vi "Dequeue Message.vi"(11 "channel":T1) -> (0 "channel aborted":bool, 1 "message data":variant, 2 "message":string)   [LabVIEW 2020, in "Message Queue.lvlib"]
doc: "This VI takes messages out of the messenger channel."
uses:
  Message Queue.lvlib
  <extravilib>/ChannelInstances/Messenger-t'Message Queue.lvlib-Message Cluster.ctl'/))Channel.ctl
  Message Cluster.ctl
  <extravilib>/ChannelInstances/Messenger-t'Message Queue.lvlib-Message Cluster.ctl'/Endpoint.vi
  <extravilib>/ChannelInstances/Messenger-t'Message Queue.lvlib-Message Cluster.ctl'.lvlib
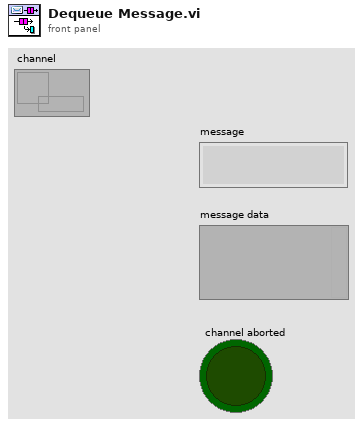
[diagram p1: front panel]
types:
  T1 = typedef "Messenger-t'Message Queue.lvlib-Message Cluster.ctl'.lvlib/))Channel.ctl" = refnum<queue>
  T2 = typedef "Message Queue.lvlib/Message Cluster.ctl" = cluster{"Message":string, "Message Data":variant}
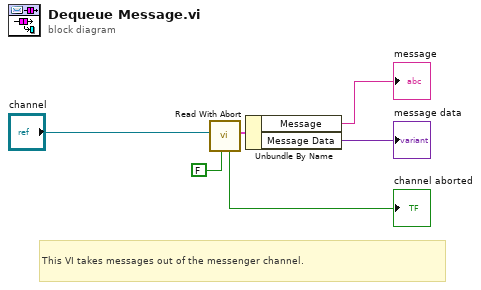
[diagram p0: block diagram]
diagram:
  # "This VI takes messages out of the messenger channel."
  n1 = call <extravilib>:"Read With Abort.vi"("abort (F)"=FALSE, "channel"="channel") -> ("element"=w6:T2, "aborted?"=→"channel aborted":bool)  [unwired: 6 in, 2 out]
  n2 = Unbundle By Name(w6) -> ("Message"=→"message":string, "Message Data"=→"message data":variant)
